vi "VisionAlign.vi"() -> ()   [LabVIEW 2018]
uses:
  Framework/Robot Global Data.vi
panel:
  in  "NoWait":bool
  in  "StoppingDistance":dbl
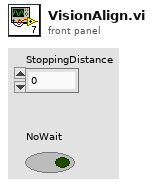
[diagram p1: front panel]
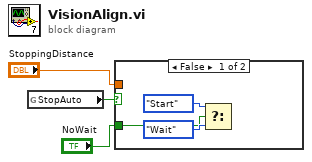
[diagram p0: block diagram]
diagram:
  n1 = global read "Robot Global Data.vi" "StopAuto"() -> (w3:bool)
  n2 = case shown="False" w3 {
    tunnel: "StoppingDistance" -> [_ _]
    tunnel: "NoWait" -> [w4 _]
    frame False {
      n3 = Select(t=enum16{"Start", "Wait"}."Start" ("Synchronization"), s=w4, f=enum16{"Start", "Wait"}."Wait" ("Synchronization")) -> ()  [unwired: 1 out]
    }
    frame True {
    }
  }
